vi "Get User Interface VI.vi"(8 "error in (no error)":errorcluster, 11 "UDP Transfer Rx User Interface in":refnum<class "UDP Transfer Rx User Interface.lvclass">) -> (0 "error out":errorcluster, 2 "user interface vi":refnum<vi>, 3 "UDP Transfer Rx User Interface out":refnum<class "UDP Transfer Rx User Interface.lvclass">)   [LabVIEW 2017, in "UDP.lvlib" / "UDP Transfer Rx User Interface.lvclass"]
uses:
  UDP Transfer Rx User Interface.lvclass
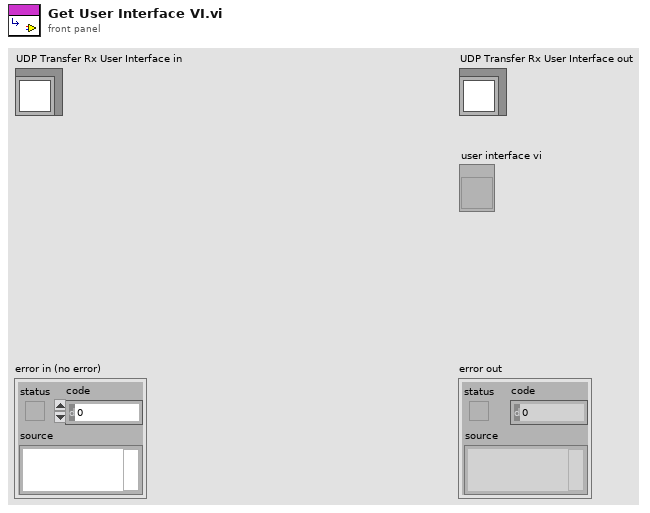
[diagram p1: front panel]
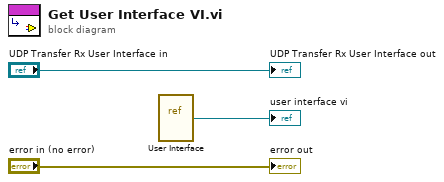
[diagram p0: block diagram]
diagram:
  n1 = vi-ref "User Interface.vi"() -> (→"user interface vi":refnum<vi>)
  "error out" <- "error in (no error)"
  "UDP Transfer Rx User Interface out" <- "UDP Transfer Rx User Interface in"
